vi "Decommit.vi"(8 "error in (no error)":errorcluster, 11 "Driver in":refnum<class "Driver.lvclass">) -> (0 "error out":errorcluster, 3 "Driver out":refnum<class "Driver.lvclass">)   [LabVIEW 2023, in "HAF.lvlib" / "Driver.lvclass"]
doc: "Set the status of all Driver Settings for this Driver to not applied."
uses:
  Driver.lvclass
  DriverSetting/DriverSetting.lvclass
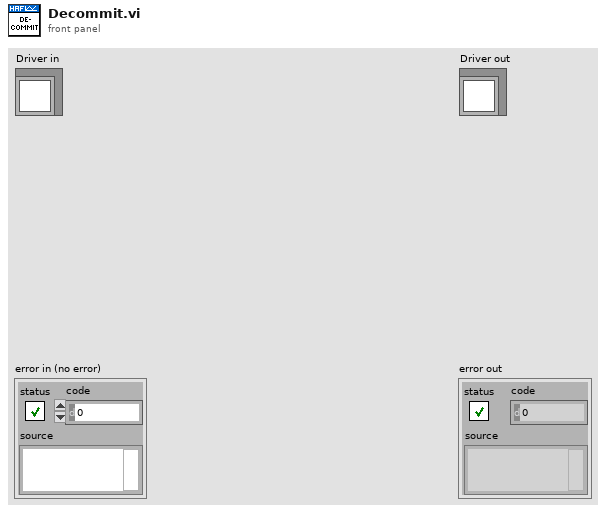
[diagram p1: front panel]
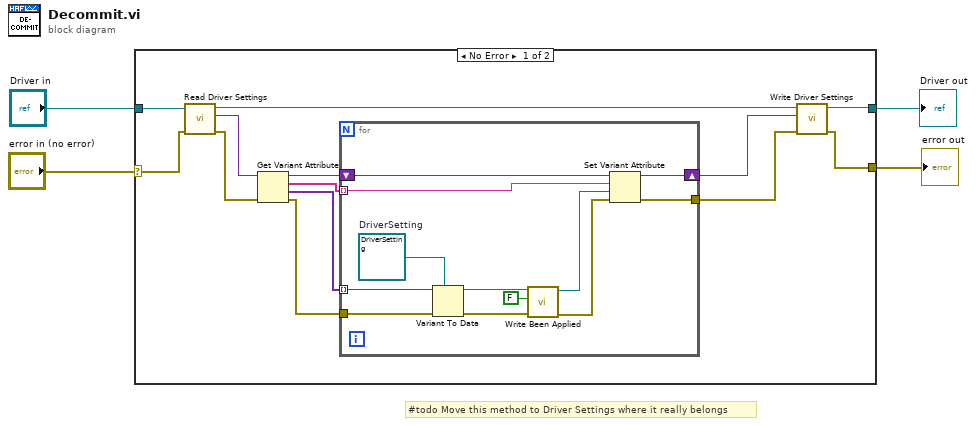
[diagram p0: block diagram]
diagram:
  # "#todo Move this method to Driver Settings where it really belongs"
  n1 = case shown="No Error" "error in (no error)" {
    selector: "error in (no error)" -> [w16 w31]
    tunnel: [w5 w31] -> w3
    tunnel: [w6 w30] -> w1
    tunnel: "Driver in" -> [w17 w30]
    frame No Error {
      n2 = call-dynamic "Read Driver Settings.vi"("error in (no error)"=w16, "Driver in"=w17) -> ("error out"=w15:errorcluster, "Driver Settings"=w14:variant, "Driver out"=w9:refnum<class "Driver.lvclass">)  [unwired: 7 in]
      n3 = Get Variant Attribute(Variant=w14, error in=w15) -> (duplicate Variant=w13:variant, names=w12:string[], values=w11:variant[], error out=w10:errorcluster)  [unwired: 2 in]
      n4 = for {
        shift-right: [w19] -> w8
        shift-left: w13 -> [w23]
        tunnel: w12 -> [w22] mode=indexing
        tunnel: w11 -> [w29] mode=indexing
        tunnel: w10 -> [w28]
        tunnel: [w18] -> w7
        w27 = refnum<class "DriverSetting.lvclass"> refnum  # DriverSetting
        n5 = Variant To Data(error in=w28, type=w27, Variant=w29) -> (data=w26:refnum<class "DriverSetting.lvclass">, error out=w24:errorcluster)
        n6 = call-dynamic "Write Been Applied.vi"("error in (no error)"=w24, "Been Applied"=FALSE, "DriverSetting in"=w26) -> ("error out"=w20:errorcluster, "DriverSetting out"=w21:refnum<class "DriverSetting.lvclass">)  [unwired: 7 in]
        n7 = Set Variant Attribute(Variant=w23, name=w22, value=w21, error in=w20) -> (Variant out=w19:variant, error out=w18:errorcluster)  [unwired: 1 out]
      }
      n8 = call-dynamic "Write Driver Settings.vi"("error in (no error)"=w7, "Driver Settings"=w8, "Driver in"=w9) -> ("error out"=w5:errorcluster, "Driver out"=w6:refnum<class "Driver.lvclass">)  [unwired: 7 in]
    }
    frame Error {
    }
  }
  "error out" <- w3
  "Driver out" <- w1
